vi "NI9237_ForceInputs_v2.vi"() -> ()   [LabVIEW 2025]
uses:
  <vilib>/DAQmx/read.llb/DAQmx Read (Analog 1D Wfm NChan NSamp).vi
  <vilib>/DAQmx/configure/timing.llb/DAQmx Timing (Sample Clock).vi
  <vilib>/DAQmx/miscellaneous.llb/DAQmx Fill In Error Info.vi
panel:
  out "error out":errorcluster
  in  "stop":bool
  out "TC2 - Inlet Thermocouple":dynamicdata(graph)
  out "LC1 - Load Cell Right":dynamicdata(graph)
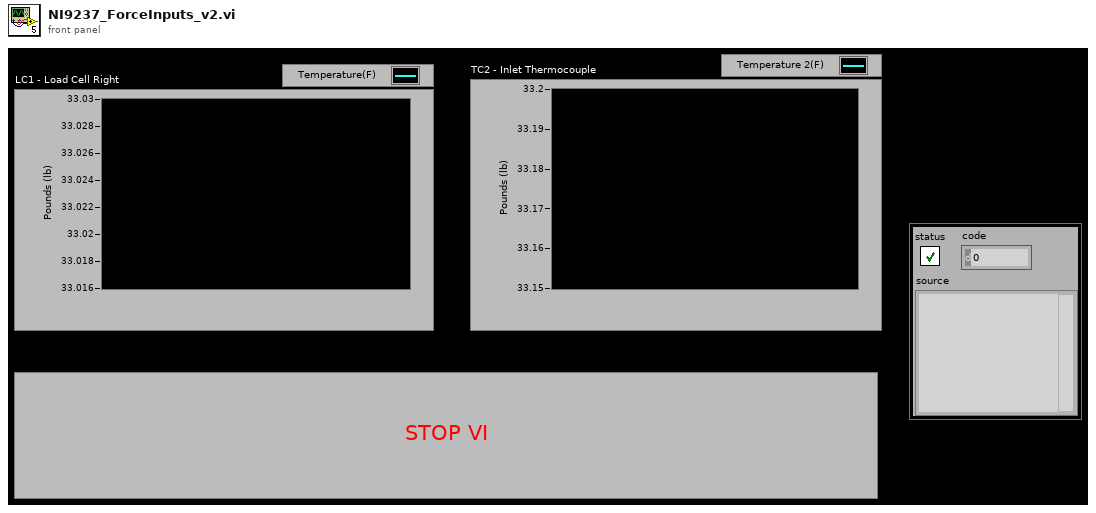
[diagram p1: front panel]
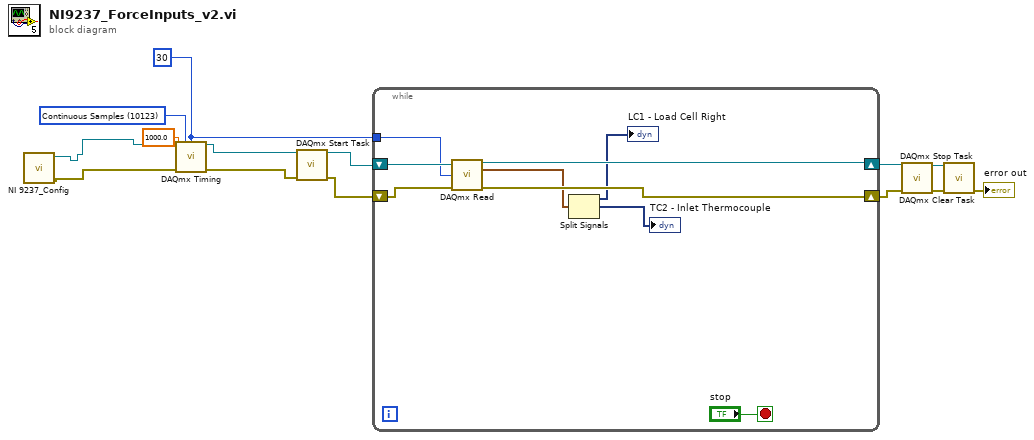
[diagram p0: block diagram]
diagram:
  w9 = 30 ("samples per channel")
  w14 = 10123 items=["Finite Samples"=10178, "Continuous Samples"=10123, "Hardware Timed Single Point"=12522] ("sample mode")
  n1 = call "NI 9237_Config.vi"() -> ("error out"=w6:errorcluster, "task out"=w7:refnum<k21>)  [unwired: 10 in]
  n2 = call-poly <vilib>:"DAQmx Timing.vi"("task/channels in"=w7, "sample mode"=w14, "samples per channel"=w9, "rate"=1000.0, "error in"=w6) -> ("task out"=w13:refnum<k21>, "error out"=w12:errorcluster)  [unwired: 9 in]
  n3 = call <vilib>:"DAQmx Start Task.vi"("task/channels in"=w13, "error in"=w12) -> ("task out"=w11:refnum<k21>, "error out"=w10:errorcluster)  [unwired: 12 in]
  n4 = while {
    shift-right: [w20] -> w3
    shift-left: w11 -> [w23]
    shift-right: [w19] -> w2
    shift-left: w10 -> [w22]
    tunnel: w9 -> [w21]
    stop <- "stop" stop-if-true
    n5 = call-poly <vilib>:"DAQmx Read.vi"("task/channels in"=w23, "number of samples per channel"=w21, "error in"=w22) -> ("task out"=w20:refnum<k21>, "data"=w18:waveform(dbl)[], "error out"=w19:errorcluster)  [unwired: 10 in]
    n6 = Split Signals(w18) -> (→"LC1 - Load Cell Right":dynamicdata, →"TC2 - Inlet Thermocouple":dynamicdata)  [unwired: 3 in, 1 out]
  }
  n7 = call <vilib>:"DAQmx Stop Task.vi"("task/channels in"=w3, "error in"=w2) -> ("task out"=w4:refnum<k21>, "error out"=w5:errorcluster)  [unwired: 12 in]
  n8 = call <vilib>:"DAQmx Clear Task.vi"("task in"=w4, "error in"=w5) -> ("error out"=→"error out":errorcluster)  [unwired: 13 in]
